vi "Scan DQMH Modules and create Maps.vi"(4 "All":bool, 6 "TreeControl in":refnum<vi>, 7 "Data Cluster In":T1, 8 "error in":errorcluster, 9 "Include Dependencies":bool, 10 "Target Selection":string, 11 "Project":string) -> (0 "error out":errorcluster, 5 "Data Cluster Out":T1={"Maps"={"Tree Map"={}, "References Map"={}}, "DQMH Scan Results"={"All DQMH Modules Refs"=[], "All Modules Descriptions"=[], "All Modules type"=[], "Project References"={"Project Ref"=refnum, "Project Name"="", "Target"=refnum, "App Ref"=refnum}, "Dependencies"=[]}, "Current Selection"={"VI Ref"=refnum, "DQMH Lib Ref"=refnum}, "Module type"=enum."Module type: Singleton", "Module ID"=-1, "Theme"=FALSE, "Broadcast?"=FALSE})   [LabVIEW 2021, in "Panther Dashboard.lvlib"]
doc: "Gets the Singleton and Cloneable references and creates a list of each type of DQMH Modules"
uses:
  Panther Dashboard.lvlib
  Module Data--cluster.ctl
  Maps List and refs--cluster.ctl
  <vilib>/National Instruments/Tree Map/Tree Map Data.ctl
  DQMH Modules Info--cluster.ctl
  Module type--enum.ctl
  Project References--cluster.ctl
  <vilib>/National Instruments/Tree Map/API/List Roots.vi
  <vilib>/National Instruments/Tree Map/Utility/Into Tree Control Items.vi
  <vilib>/Delacor/Delacor QMH/Libraries/Scripting API/DQMH_Scripting API.lvlib
  <vilib>/National Instruments/Tree Map/Tree Map.lvlib
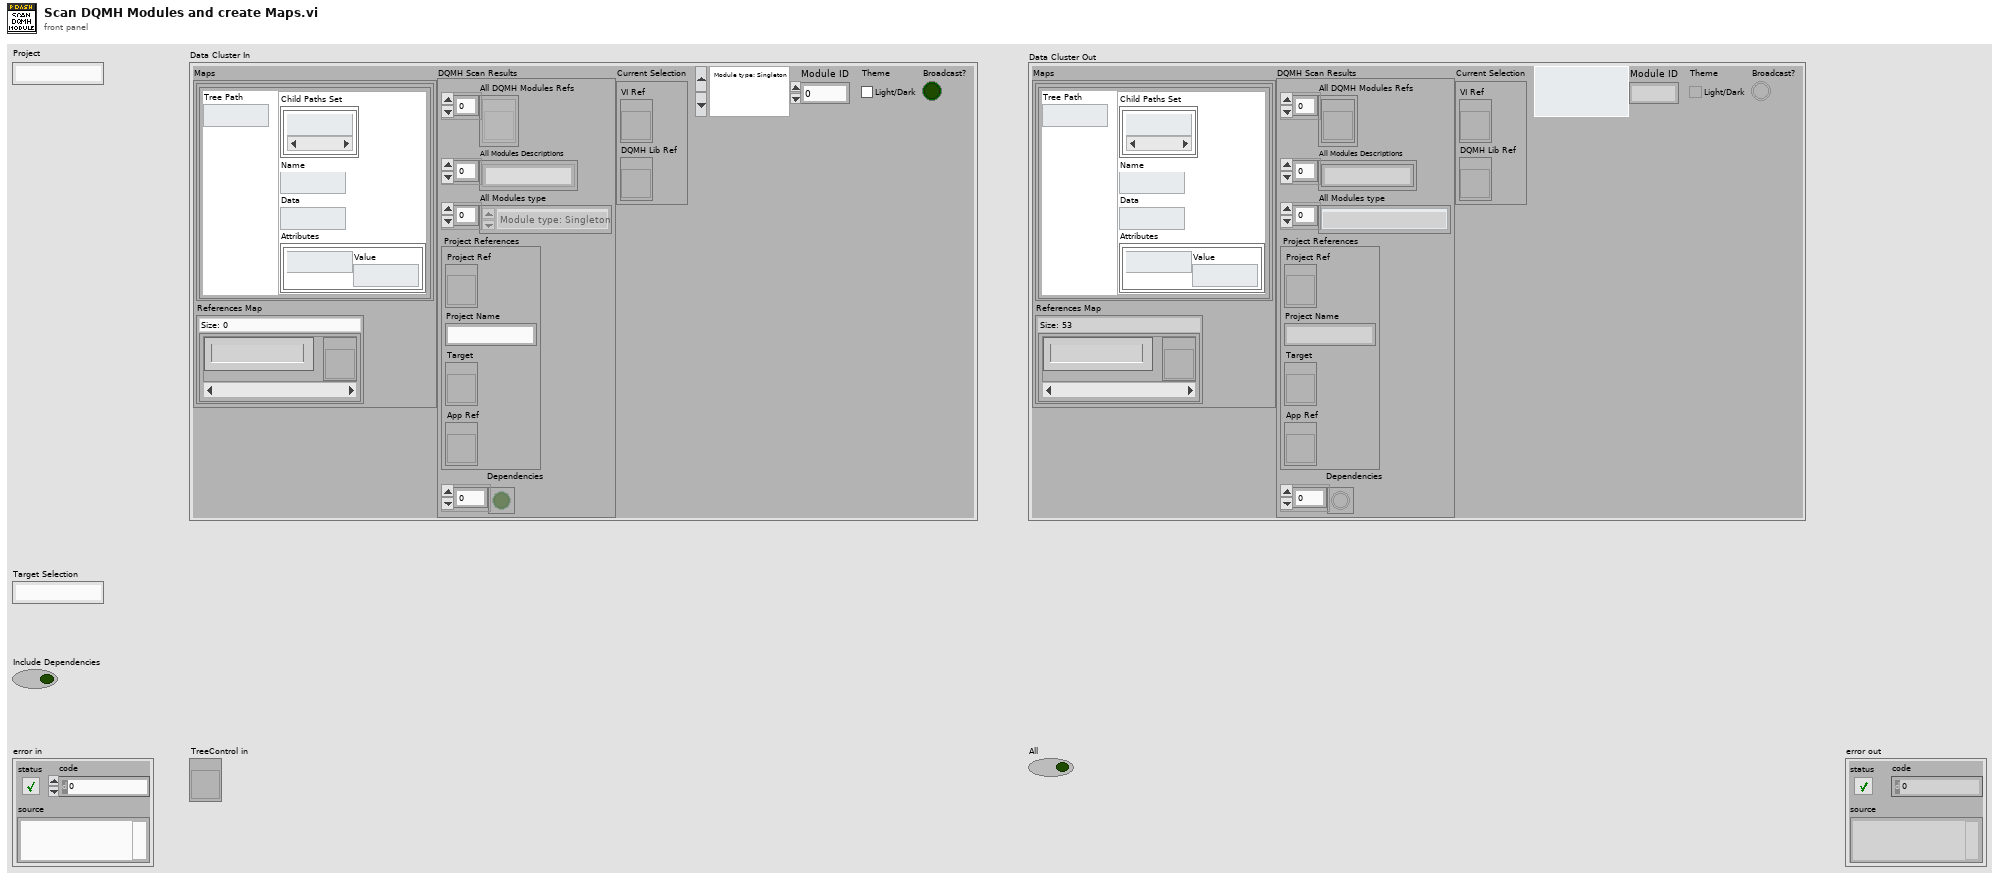
[diagram p1: front panel]
types:
  T1 = typedef "Panther Dashboard.lvlib/Module Data--cluster.ctl" = cluster{"Maps":T2, "DQMH Scan Results":T4, "Current Selection":cluster{"VI Ref":refnum<vi>, "DQMH Lib Ref":refnum<vi>}, "Module type":T5, "Module ID":i32, "Theme":bool, "Broadcast?":bool}
  T2 = typedef "Panther Dashboard.lvlib/Maps List and refs--cluster.ctl" = cluster{"Tree Map":T3, "References Map":map{string, refnum<vi>}}
  T3 = typedef "Tree Map.lvlib/Tree Map Data.ctl" = map{string, cluster{"Child Paths Set":set{string}, "Name":string, "Data":string, "Attributes":map{string, string}}}
  T4 = typedef "Panther Dashboard.lvlib/DQMH Modules Info--cluster.ctl" = cluster{"All DQMH Modules Refs":refnum<vi>[], "All Modules Descriptions":string[], "All Modules type":T5[], "Project References":T6, "Dependencies":bool[]}
  T5 = typedef "Panther Dashboard.lvlib/Module type--enum.ctl" = enum16{"Module type: Singleton", "Module type: Cloneable"}
  T6 = typedef "Panther Dashboard.lvlib/Project References--cluster.ctl" = cluster{"Project Ref":refnum<vi>, "Project Name":string, "Target":refnum<vi>, "App Ref":refnum<vi>}
  T7 = typedef "DQMH_Scripting API.lvlib/Module Information--cluster.ctl" = cluster{"Library":refnum<vi>, "Qualified Name":string, "Path":path, "Cloneable":bool, "Under Dependencies":bool}
  T8 = cluster{"Left Cell String":string, "Child Text":string[], "Child Tag":string, "Item Indent":i32, "Child Only?":bool, "Glyph Index":i32}[]
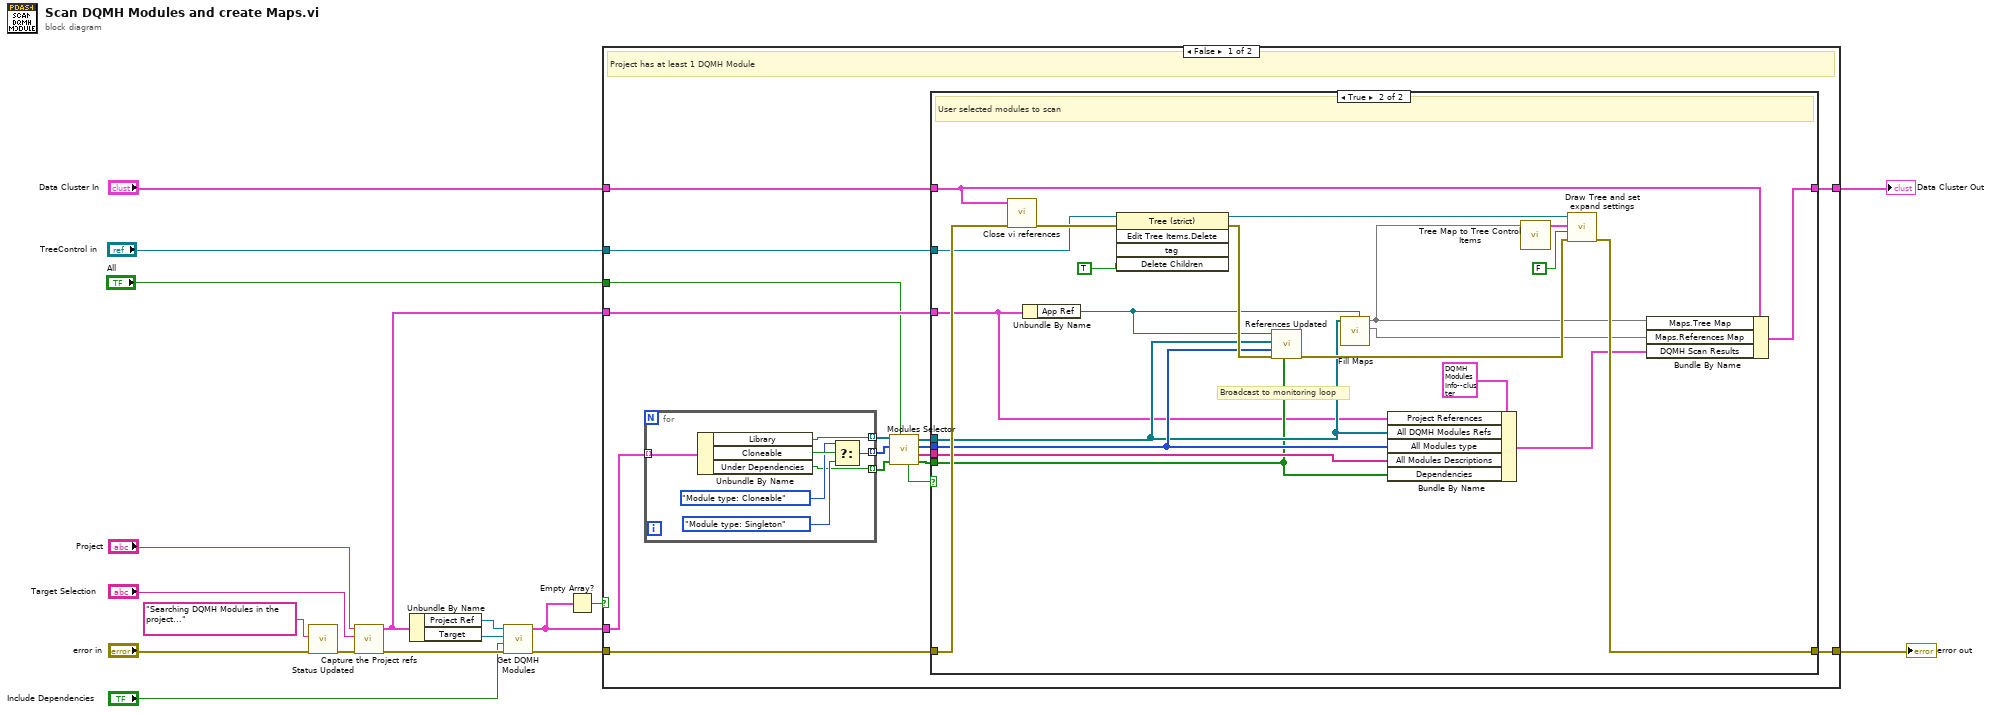
[diagram p0: block diagram]
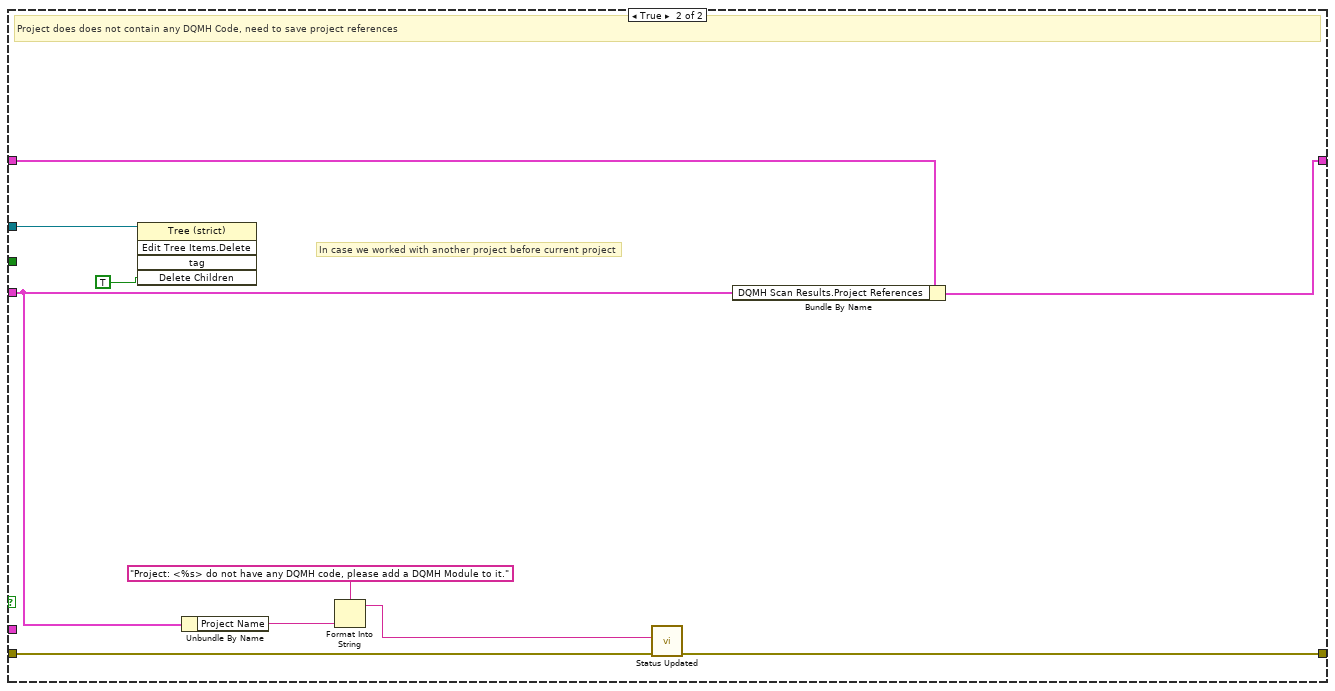
[diagram p3: hidden frame]
diagram:
  n1 = call "Status Updated.vi"("error in (no error)"="error in", "Status"="Searching DQMH Modules in the project...") -> ("error out"=w16:errorcluster)  [unwired: 9 in]
  n2 = call "Capture the Project refs.vi"("error in"=w16, "Target Selection"="Target Selection", "Project Selection"="Project") -> ("error out"=w18:errorcluster, "References"=w7:T6)  [unwired: 7 in]
  n3 = Unbundle By Name(w7) -> ("Project Ref"=w9:refnum<vi>, "Target"=w8:refnum<vi>)
  n4 = call <vilib>:"Get DQMH Modules.vi"("error in"=w18, "Include Dependencies (F)"="Include Dependencies", "Target (My Computer)"=w8, "Project"=w9) -> ("error out"=w15:errorcluster, "DQMH Modules"=w2:T7[])  [unwired: 6 in]
  n5 = Empty Array?(array=w2) -> (empty?=w3:bool)
  n6 = case shown="False" w3 {
    tunnel: w15 -> [w34 w75]
    tunnel: [w33 w72] -> w14
    tunnel: w7 -> [w29 w71]
    tunnel: "Data Cluster In" -> [w27 w74]
    tunnel: [w26 w73] -> w5
    tunnel: "TreeControl in" -> [w24 w66]
    tunnel: w2 -> [w23 _]
    tunnel: "All" -> [w19 _]
    frame False {
      # "Project has at least 1 DQMH Module"
      n7 = for {
        tunnel: w23 -> [w65] mode=indexing
        tunnel: [w64] -> w22 mode=indexing
        tunnel: [w60] -> w21 mode=indexing
        tunnel: [w59] -> w20 mode=indexing
        n8 = Unbundle By Name(w65) -> ("Library"=w64:refnum<vi>, "Cloneable"=w62:bool, "Under Dependencies"=w59:bool)
        n9 = Select(t=Module_type--enum."Module type: Cloneable", s=w62, f=Module_type--enum."Module type: Singleton" ("Module type")) -> (s? t:f=w60:T5)
      }
      n10 = call "Modules Selector.vi"("Scan All"=w19, "Module In Dependencies?"=w20, "Modules Types In"=w21, "DQMH Modules In"=w22) -> ("Module In Dependencies?Out"=w28:bool[], "Descriptions"=w32:string[], "Modules Types Out"=w31:T5[], "DQMH Modules Out"=w30:refnum<vi>[], "Scan?"=w25:bool)  [unwired: 3 in]
      n11 = case shown="True" w25 {
        tunnel: w32 -> [_ w52]
        tunnel: w31 -> [_ w50]
        tunnel: w30 -> [_ w49]
        tunnel: w29 -> [_ w37]
        tunnel: w28 -> [_ w48]
        tunnel: w27 -> [w35 w44]
        tunnel: [w35 w45] -> w26
        tunnel: w24 -> [_ w41]
        tunnel: w34 -> [w36 w56]
        tunnel: [w36 w54] -> w33
        frame False {
          # "User Cancel Scan process, do not redraw tree and keep previous selection"
        }
        frame True {
          # "Broadcast to monitoring loop"
          # "User selected modules to scan"
          n12 = call "Close vi references.vi"("error in"=w56, "Data Cluster"=w44) -> ("error out"=w58:errorcluster)  [unwired: 9 in]
          n13 = Unbundle By Name(w37) -> ("App Ref"=w51:refnum<vi>)
          n14 = invoke class="Tree (strict)" method="Edit Tree Items.Delete"(reference=w41, error in=w58, "Delete Children"=TRUE ("Delete Children?")) -> (reference out=w39:refnum<vi>, error out=w57:errorcluster)  [unwired: 2 in, 3 out]
          n15 = call "References Updated.vi"("Dependencies"=w48, "error in"=w57, "Modules Types"=w50, "Modules"=w49, "Application Instance"=w51) -> ("error out"=w55:errorcluster)  [unwired: 6 in]
          n16 = call "Fill Maps.vi"("App Ref"=w51, "DQMH Modules"=w49) -> ("map ref out"=w47:map{string, refnum<vi>}, "Tree Map out"=w42:T3)  [unwired: 8 in]
          n17 = Bundle By Name(cluster=T4 {"All DQMH Modules Refs"=[], "All Modules Descriptions"=[], "All Modules type"=[], "Project References"={"Project Ref"=refnum, "Project Name"="", "Target"=refnum, "App Ref"=refnum}, "Dependencies"=[]} ("DQMH Scan Results"), "Project References"=w37, "All DQMH Modules Refs"=w49, "All Modules type"=w50, "All Modules Descriptions"=w52, "Dependencies"=w48) -> (w46:T4)
          n18 = call <vilib>:"Tree Map to Tree Control Items.vi"("Tree Map In"=w42) -> ("Tree Control Items"=w43:T8)  [unwired: 10 in]
          n19 = call "Draw Tree and set expand settings.vi"("error in"=w55, "Expanded Results?"=FALSE, "Tree Control Items"=w43, "TreeControl in"=w39) -> ("error out"=w54:errorcluster)  [unwired: 7 in]
          n20 = Bundle By Name(cluster=w44, "Maps.Tree Map"=w42, "Maps.References Map"=w47, "DQMH Scan Results"=w46) -> (w45:T1)
        }
      }
    }
    frame True {
      # "In case we worked with another project before current project"
      # "Project does does not contain any DQMH Code, need to save project references"
      n21 = invoke class="Tree (strict)" method="Edit Tree Items.Delete"(reference=w66, "Delete Children"=TRUE ("Delete Children?")) -> ()  [unwired: 3 in, 5 out]
      n22 = Unbundle By Name(w71) -> ("Project Name"=w70:string)
      n23 = Format Into String(format string="Project: <%s> do not have any DQMH code, please add a DQMH Module to it.", w70) -> (resulting string=w69:string)  [unwired: 2 in, 1 out]
      n24 = call "Status Updated.vi"("error in (no error)"=w75, "Status"=w69) -> ("error out"=w72:errorcluster)  [unwired: 9 in]
      n25 = Bundle By Name(cluster=w74, "DQMH Scan Results.Project References"=w71) -> (w73:T1)
    }
  }
  "error out" <- w14
  "Data Cluster Out" <- w5
